vi "Read from PGSQL (unused).vi"(8 "error in (no error)":errorcluster, 10 "path":string, 11 "Logger in":refnum<class "Logger.PGSQL.lvclass">) -> (0 "error out":errorcluster, 1 "Variant":variant, 3 "Logger out":refnum<class "Logger.PGSQL.lvclass">)   [LabVIEW 2016, in "Logger.PGSQL.lvclass"]
uses:
  Logger.PGSQL.lvclass
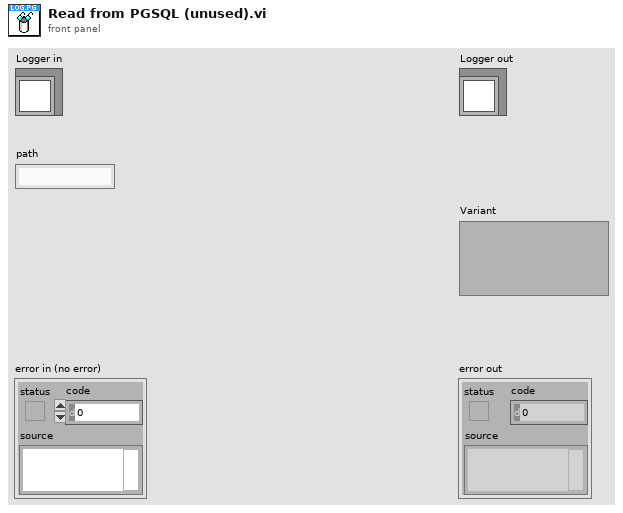
[diagram p1: front panel]
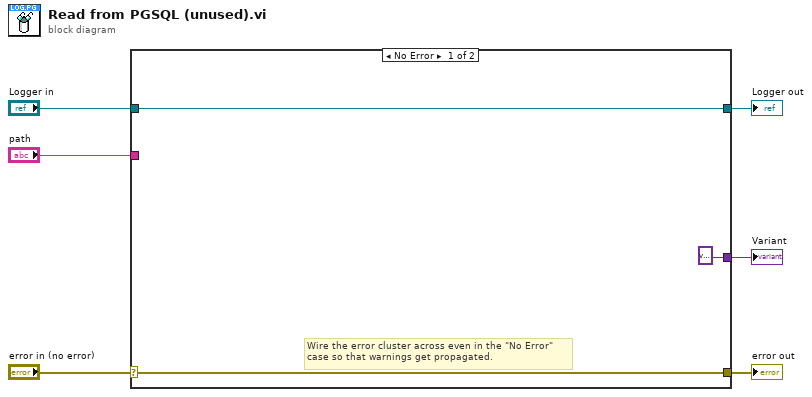
[diagram p0: block diagram]
diagram:
  n1 = case shown="No Error" "error in (no error)" {
    selector: "error in (no error)" -> [w8 w11]
    tunnel: [w8 w11] -> w5
    tunnel: [w9 w10] -> w3
    tunnel: "Logger in" -> [w9 w10]
    tunnel: "path" -> [_ _]
    tunnel: [variant ("Variant") _] -> w1
    frame No Error {
      # "Wire the error cluster across even in the \"No Error\"\ncase so that warnings get propagated."
    }
    frame Error {
    }
  }
  "error out" <- w5
  "Logger out" <- w3
  "Variant" <- w1
